vi "IDS_axis_getPassMode.vi"(8 "error in (no error)":errorcluster, 11 "deviceHandle":i32) -> (0 "error out":errorcluster, 2 "mode out":i32, 3 "deviceHandle out":i32)   [LabVIEW 2016]
doc: "int IDS_DLL IDS_axis_getPassMode(int32_t * mode);"
panel:
  in  "mode":i32
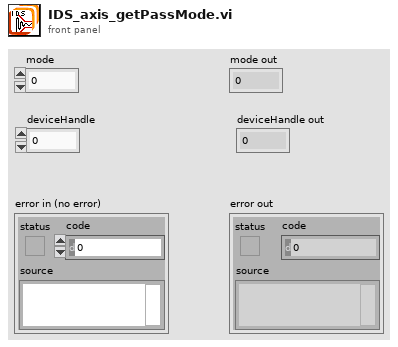
[diagram p1: front panel]
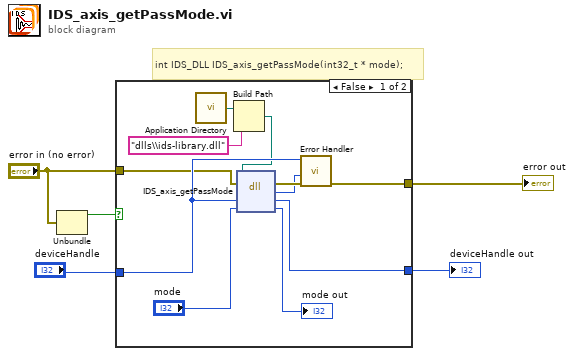
[diagram p0: block diagram]
diagram:
  # "int IDS_DLL IDS_axis_getPassMode(int32_t * mode);"
  n1 = Unbundle("error in (no error)") -> ("status"=w1:bool)  [unwired: 2 out]
  n2 = case shown="False" w1 {
    tunnel: [w16 w17] -> w5
    tunnel: "deviceHandle" -> [w10 w18]
    tunnel: [w12 w18] -> w3
    tunnel: "error in (no error)" -> [w9 w17]
    frame False {
      n3 = call <vilib>:"Application Directory.vi"() -> ("Application Directory"=w8:path)
      n4 = Build Path(base path=w8, name or relative path="dlls\\ids-library.dll" ("ipAddress")) -> (appended path=w6:path)
      n5 = dll-call lib="C:/Users/matheus/Desktop/LabVIEW_Draft_V1.6.0/dlls/ids-library.*" fn="IDS_axis_getPassMode"(path in=w6, error in=w9, "deviceHandle"=w10, "mode"="mode") -> (error out=w15:errorcluster, "Rückgabetyp"=w11:i32, "deviceHandle"=w12:i32, "mode"=→"mode out":i32)  [unwired: 1 in, 1 out]
      n6 = call "Error Handler.vi"("error in (no error)"=w15, "error code"=w11, "deviceHandle"=w10) -> ("error out"=w16:errorcluster)  [unwired: 7 in, 1 out]
    }
    frame True {
    }
  }
  "error out" <- w5
  "deviceHandle out" <- w3
